vi "SF2 Save Orentation History .vi"(11 "Loop Frequency (msec)":u32) -> ()   [LabVIEW 2016]
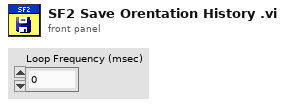
[diagram p1: front panel]
types:
  T1 = typedef "SF2_NotifyPacketTypeDef.ctl" = cluster{"SF2 Action":T2, "Data":variant}
  T2 = typedef "SF2_ActionTypeDef.ctl" = enum16{"None", "Halt", "Start Recording", "Stop Recording", "Reset Buffer"}
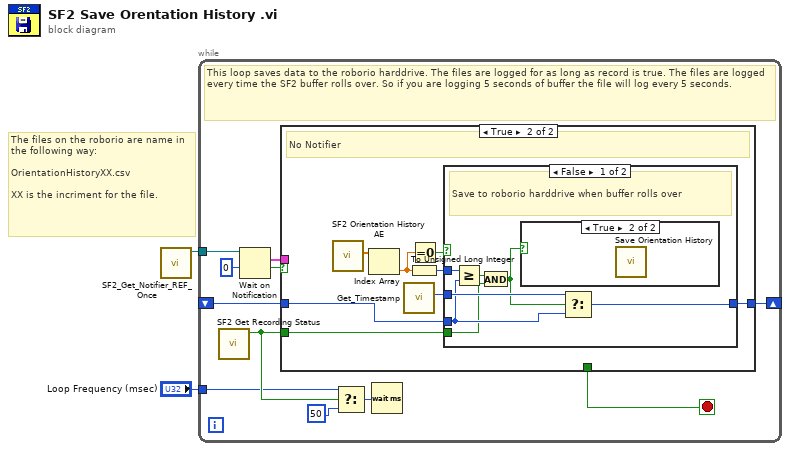
[diagram p0: block diagram]
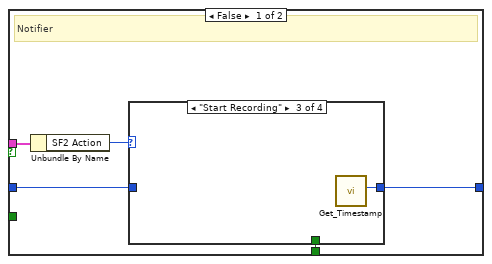
[diagram p2: hidden frame]
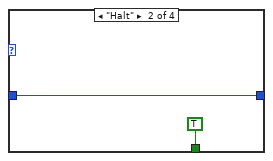
[diagram p4: hidden frame]
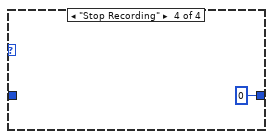
[diagram p5: hidden frame]
diagram:
  # "The files on the roborio are name in the following way:\n\nOrientationHistoryXX.csv\n\nXX is the incriment for the file."
  n1 = call "SF2_Get_Notifier_REF_Once.vi"() -> ("notifier ref out"=w2:refnum<notifier>)  [unwired: 10 in, 1 out]
  n2 = while {
    shift-right: [w13] -> _
    shift-left: _ -> [w12]
    tunnel: w2 -> [w10]
    tunnel: "Loop Frequency (msec)" -> [w3]
    stop <- w7 stop-if-true
    # "This loop saves data to the roborio harddrive. The files are logged for as long as record is true. The files are logged every time the SF2 buffer rolls over. So if you are logging 5 seconds of buffer the file will log every 5 seconds."
    n3 = call "SF2 Get Recording Status.vi"() -> ("Recording (out)"=w6:bool)  [unwired: 11 in]
    n4 = Wait on Notification(notifier=w10, timeout in ms (-1)=0) -> (notification=w8:T1, timed out?=w9:bool)  [unwired: 2 in, 2 out]
    n5 = case shown="True" w9 {
      tunnel: [w16 w31] -> w13
      tunnel: w12 -> [w15 w27]
      tunnel: w8 -> [w17 _]
      tunnel: [w14 _] -> w7
      tunnel: w6 -> [_ w24]
      frame False {
        # "Notifier"
        n6 = Unbundle By Name(w17) -> ("SF2 Action"=w18:T2)
        n7 = case shown="\"Start Recording\"" w18 {
          tunnel: [w19 w21 w22 u32 0 ("Timestamp")] -> w16
          tunnel: w15 -> [w19 w21 _ _]
          tunnel: [_ TRUE _ _] -> w14
          frame "None", Default {
          }
          frame "Halt" {
            # "Got Notifier"
          }
          frame "Start Recording" {
            n8 = call "Get_Timestamp.vi"() -> ("Timestamp"=w22:u32)  [unwired: 11 in]
          }
          frame "Stop Recording" {
          }
        }
      }
      frame True {
        # "No Notifier"
        n9 = call "SF2 Orientation History AE.vi"() -> ("deleted (out)"=w30:dbl[])  [unwired: 10 in, 1 out]
        n10 = Index Array(array=w30) -> (element=w29:dbl)  [unwired: 1 in]
        n11 = call "Get_Timestamp.vi"() -> ("Timestamp"=w28:u32)  [unwired: 11 in]
        n12 = To Unsigned Long Integer(number=w29) -> (unsigned 32bit integer=w25:u32)
        n13 = Equal To 0?(x=w29) -> (x = 0?=w26:bool)
        n14 = case shown="False" w26 {
          tunnel: w27 -> [w35 _]
          tunnel: w28 -> [w36 w39]
          tunnel: [w38 w39] -> w31
          tunnel: w25 -> [w37 _]
          tunnel: w24 -> [w32 _]
          frame False {
            # "Save to roborio harddrive when buffer rolls over"
            n15 = Greater Or Equal?(x=w37, y=w35) -> (x >= y?=w33:bool)
            n16 = And(x=w33, y=w32) -> (x .and. y?=w34:bool)
            n17 = case shown="True" w34 {
              frame False {
              }
              frame True {
                n18 = call "Save Orientation History.vi"() -> ()  [unwired: 10 in, 2 out]
              }
            }
            n19 = Select(t=w36, s=w34, f=w35) -> (s? t:f=w38:u32)
          }
          frame True {
            # "Not logging data"
          }
        }
      }
    }
    n20 = Select(t=w3, s=w6, f=u32 50) -> (s? t:f=w5:u32)
    n21 = Wait (ms)(milliseconds to wait=w5) -> ()  [unwired: 1 out]
  }
